vi "simple control.vi"() -> ()   [LabVIEW 2024]
panel:
  out "Numeric control":dbl
  in  "y":dbl
  in  "x":dbl
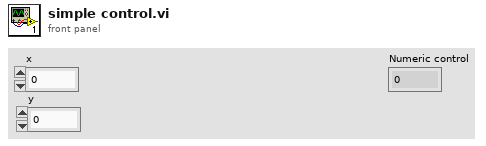
[diagram p1: front panel]
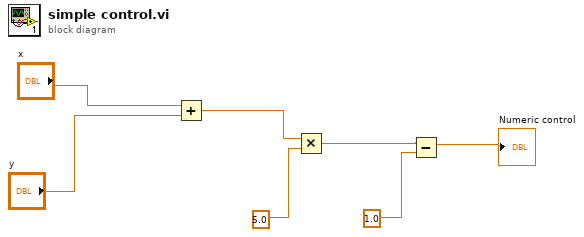
[diagram p0: block diagram]
diagram:
  n1 = Add(x="x", y="y") -> (x+y=w2:dbl)
  n2 = Multiply(x=w2, y=5.0) -> (x*y=w7:dbl)
  n3 = Subtract(x=w7, y=1.0) -> (x-y=→"Numeric control":dbl)
